vi "Backup File.vi"(10 "列首字符串":string[](array[string]), 11 "path":path) -> (3 "path 2":path)   [LabVIEW 2017]
uses:
  <vilib>/Utility/file.llb/Read Delimited Spreadsheet (string).vi
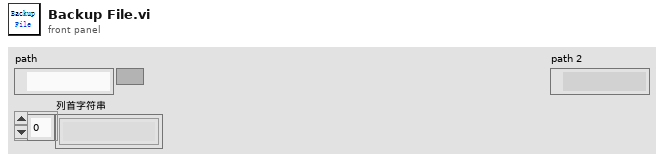
[diagram p1: front panel]
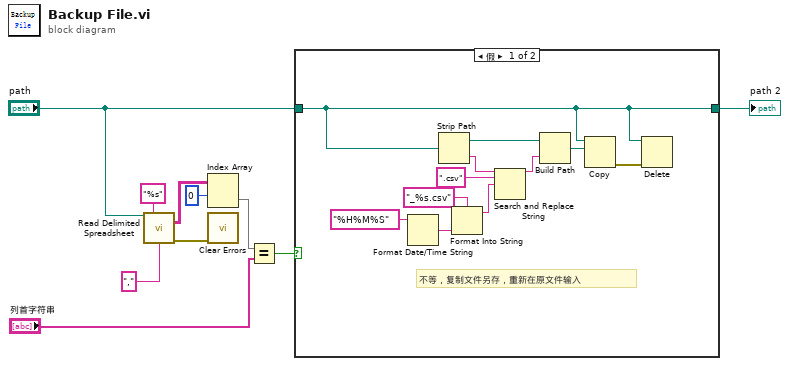
[diagram p0: block diagram]
diagram:
  n1 = call-poly <vilib>:"Read Delimited Spreadsheet.vi"("file path (dialog if empty)"="path", "format (%s)"="%s", "delimiter (\\t)"="," ("format (%s)")) -> ("all rows"=w3:string[][], "error out"=w5:errorcluster)  [unwired: 7 in, 4 out]
  n2 = Index Array(array=w3, index (row)=0 ("索引 (行)")) -> (element=w6:string[])  [unwired: 1 in]
  n3 = call <vilib>:"Clear Errors.vi"("error in (no error)"=w5) -> ()  [unwired: 5 in, 2 out]
  n4 = Equal?(x=w6, y="列首字符串") -> (x = y?=w1:bool)
  n5 = case shown="假" w1 {
    tunnel: [w21 w22] -> w2
    tunnel: "path" -> [w21 w22]
    frame False {
      # "不等，复制文件另存，重新在原文件输入"
      n6 = Format Date/Time String(time format string (%c)="%H%M%S" ("时间格式字符串(%c)")) -> (date/time string=w13:string)  [unwired: 2 in]
      n7 = Strip Path(path=w21) -> (stripped path=w19:path, name=w20:string)
      n8 = Format Into String(format string="_%s.csv" ("格式字符串"), w13) -> (resulting string=w16:string)  [unwired: 2 in, 1 out]
      n9 = Search and Replace String(input string=w20, search string=".csv" ("时间格式字符串(%c)"), replace string=w16) -> (result string=w18:string)  [unwired: 5 in, 3 out]
      n10 = Build Path(base path=w19, name or relative path=w18) -> (appended path=w12:path)
      n11 = Copy(10:w12, 11:w21) -> (0:w11:errorcluster)  [unwired: 3 in, 2 out]
      n12 = Delete(path (use dialog)=w21, error in=w11) -> ()  [unwired: 3 in, 3 out]
    }
    frame True {
      # "表头相等，原路径"
    }
  }
  "path 2" <- w2
